vi "Set Exposure Mode.vi"(8 "error in (no error)":errorcluster, 10 "exposure mode":T1=enum."automatic") -> (0 "error out":errorcluster, 2 "return value":i32)   [LabVIEW 2009, in "HighFinesse WS5.lvlib"]
doc: "Sets the exposure mode of the wavelength meter to either manual or automatic."
uses:
  HighFinesse WS5.lvlib
  Variable Typedefs.llb/Exposure Mode.ctl
  WINDOWS/system32/wlmData.dll
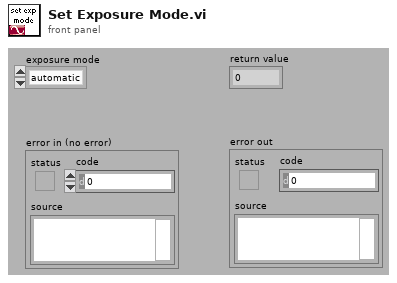
[diagram p1: front panel]
types:
  T1 = typedef "HighFinesse WS5.lvlib/Exposure Mode.ctl" = enum16{"manual", "automatic"}
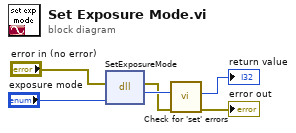
[diagram p0: block diagram]
diagram:
  n1 = dll-call lib="C:/WINDOWS/system32/wlmData.dll" fn="SetExposureMode"(error in="error in (no error)", "EM"="exposure mode") -> (error out=w4:errorcluster, "return value"=w6:i32)  [unwired: 2 in, 2 out]
  n2 = call "Check for 'set' errors.vi"("error in (no error)"=w4, "return value"=w6) -> ("error out"=→"error out":errorcluster, "return value out"=→"return value":i32)  [unwired: 8 out]
